vi "Close-Power.vi"(8 "error in (no error)":errorcluster) -> ()   [LabVIEW 2014]
uses:
  Global variables.vi
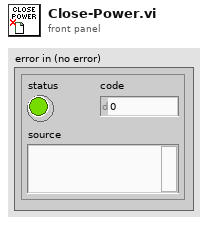
[diagram p1: front panel]
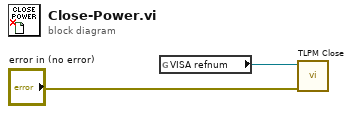
[diagram p0: block diagram]
diagram:
  n1 = global read "Global variables.vi" "VISA refnum"() -> (w1:refnum<visa-resource-name>)
  n2 = call <instrlib>:"TLPM Close.vi"("error in (no error)"="error in (no error)", "instrument handle"=w1) -> ()  [unwired: 9 in, 1 out]
